vi "single fit V4 - rec.vi"(5 "cursor bracket: fragment  ref":refnum<vi>, 6 "main VI path":path, 7 "factor":dbl=7.0, 8 "pond":cdb[][](array[numeric]), 9 "wave packet":cdb[][](array[numeric]), 10 "omega map parameters":T2={"map method"=enum."less trivial", "2:window factor"=1, "left"=3.0, "right"=3.0, "omega"=3.0, "gamma"=3.0, "theta0"=3.0, "use points"=enum."decimated", "z(inf) method"=enum."median"}, 11 "single fit parameters":T3={"number of 2D grid points"=300, "# of points in pond"=339, "# of points in window"=10919, "decimation threshold"=1, "normalization factor"=0.029014793, "pond scale factor "=3.0, "normalized z"=[], "decimated z"=[], "decimated omega"=[], "omega in window"=[], "z in window"=[], "data center"=3.0+0.0i, "inverse"=[], "linear "=[], "omega around"=[], "phase around center"=[], "fit for phase around senter "=[], "three points"={[], []}, "max omega"=0.029014793, "min omega"=0.029014793}) -> (0 "lorentzian out":T5={"Amplitude"=-1.0311345636926572, "omega(0)"=-1.0311345636926572, "Gamma"=-1.0311345636926572, "phase"=-1.0311345636926572, "Q"=-1.0311345636926572, "Norm  Ampl"=-1.0311345636926572, "z (inf)"=-1.0311345636926572+0.0i, "4corners"={"z (-pi/2)"=-1.0311345636926572+0.5736824521422934i, "z(inf)"=-0.5200164984937075+1.0975277942502903i, "z (pi/2)"=-1.0311345636926572+0.5736824521422934i, "z center"=-0.5136528600391839+0.580046090596817i, "z(0)"=-0.5200164984937075+1.0975277942502903i, "radius"=-1.0311345636926572}} {"Q" format="%#_8f"; "phase" format="%#_6f"; "Gamma" format="%#_8f"; "omega(0)" format="%#_8f"}, 2 "omega map parameters out":T2={"map method"=enum."less trivial", "2:window factor"=1, "left"=3.0, "right"=3.0, "omega"=3.0, "gamma"=3.0, "theta0"=3.0, "use points"=enum."decimated", "z(inf) method"=enum."median"}, 3 "single fit parameters out":T3={"number of 2D grid points"=300, "# of points in pond"=339, "# of points in window"=10919, "decimation threshold"=1, "normalization factor"=0.029014793, "pond scale factor "=3.0, "normalized z"=[], "decimated z"=[], "decimated omega"=[], "omega in window"=[], "z in window"=[], "data center"=3.0+0.0i, "inverse"=[], "linear "=[], "omega around"=[], "phase around center"=[], "fit for phase around senter "=[], "three points"={[], []}, "max omega"=0.029014793, "min omega"=0.029014793}, 4 "complex region out":T4={"max re"=1.1965102077412717, "min re"=-1.8034897922587283, "max im"=1.1920568931854867, "min im"=-1.636084117505164, "delta re"=3.0, "delta im"=2.8281410106906506, "center re"=-0.3034897922587282, "delta  z"=3.0+2.8281410106906506i, "center im"=-0.2220136121598386, "center z"=-0.3034897922587282+2.8281410106906506i, "d im"=0.0, "d re"=0.0, "d z"=0.0+0.0i})   [LabVIEW 2010]
uses:
  lorentzian.ctl
  circle corners.ctl
  complex region.ctl
  single fit parameters.ctl
  omega map parameters.ctl
  cursor winow.ctl
  cursor window action.ctl
  peak - simple guess at omega.vi
  peak - less simple guess at omega.vi
  peak - fix phase.vi
  peak - fit phase around center.vi
  peak - geometry fit.vi
  find circle corners V3.vi
  peak - phase around center.vi
  peak - linear and inverse maps.vi
  peak - calculate lorentzian.vi
  index from range.vi
  <vilib>/Analysis/baseanly.llb/Mean.vi
  <vilib>/Analysis/baseanly.llb/Median.vi
  <vilib>/Analysis/2dsp.llb/Unwrap Phase.vi
  <vilib>/gmath/interp.llb/Interpolate 1D.vi
  <vilib>/gmath/NumericalOptimization/Nonlinear Curve Fit.vi
  <vilib>/gmath/NumericalOptimization/Nonlinear Curve Fit LM.vi
  <vilib>/Utility/error.llb/Clear Errors.vi
  <vilib>/Analysis/6fits.llb/Linear Fit.vi
panel:
  in  "cursor bracket in":T1={"left"=2044.0881763527054, "right "=2126.7657992565055, "center"=2085.4269878046052, "window"=82.67762290380006, "cursors"=[], "relative"=0, "absolute"=0, "fixed vertical offset"=2421.6740576496672, "vertical offset"=2421.6740576496672, "skew"=2421.6740576496672, "default window frac"=2421.6740576496672, "kind"=enum."fancy", "skew.left"=2.0, "skew.right"=0.0, "Plot ref"=refnum, "wing order"=enum."back"}
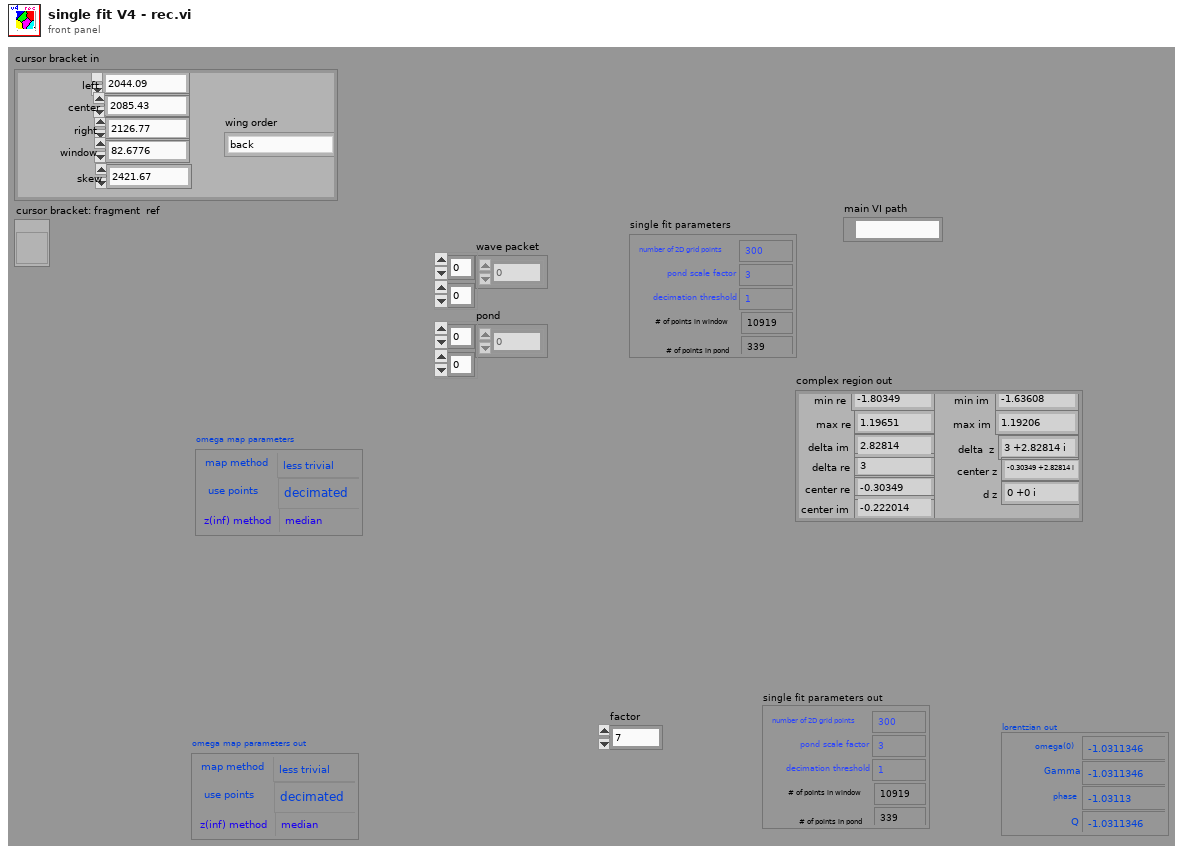
[diagram p1: front panel]
types:
  T1 = typedef "cursor winow.ctl" = cluster{"left":dbl, "right ":dbl, "center":dbl, "window":dbl, "cursors":i32[], "relative":i32, "absolute":i32, "fixed vertical offset":dbl, "vertical offset":dbl, "skew":dbl, "default window frac":dbl, "kind":enum16{"symmetric", "skewed", "fancy"}, "skew.left":dbl, "skew.right":dbl, "Plot ref":refnum<vi>, "wing order":enum16{"forw", "back"}}
  T2 = typedef "omega map parameters.ctl" = cluster{"map method":enum16{"simple", "less trivial", "around center", "geometry"}, "2:window factor":i32, "left":dbl, "right":dbl, "omega":dbl, "gamma":dbl, "theta0":dbl, "use points":enum16{"all in window", "decimated"}, "z(inf) method":enum16{"median", "method 2", "histogram"}}
  T3 = typedef "single fit parameters.ctl" = cluster{"number of 2D grid points":i32, "# of points in pond":i32, "# of points in window":i32, "decimation threshold":i32, "normalization factor":dbl, "pond scale factor ":dbl, "normalized z":cdb[], "decimated z":cdb[], "decimated omega":dbl[], "omega in window":dbl[], "z in window":cdb[], "data center":cdb, "inverse":cdb[], "linear ":cdb[], "omega around":dbl[], "phase around center":dbl[], "fit for phase around senter ":dbl[], "three points":cluster{dbl[], dbl[]}, "max omega":dbl, "min omega":dbl}
  T4 = typedef "complex region.ctl" = cluster{"max re":dbl, "min re":dbl, "max im":dbl, "min im":dbl, "delta re":dbl, "delta im":dbl, "center re":dbl, "delta  z":cdb, "center im":dbl, "center z":cdb, "d im":dbl, "d re":dbl, "d z":cdb}
  T5 = typedef "lorentzian.ctl" = cluster{"Amplitude":dbl, "omega(0)":dbl, "Gamma":dbl, "phase":dbl, "Q":dbl, "Norm  Ampl":dbl, "z (inf)":cdb, "4corners":T6}
  T6 = typedef "circle corners.ctl" = cluster{"z (-pi/2)":cdb, "z(inf)":cdb, "z (pi/2)":cdb, "z center":cdb, "z(0)":cdb, "radius":dbl}
  T7 = enum16{"simple", "less trivial", "around center", "geometry"}
  T8 = cluster{"left":dbl, "right ":dbl, "center":dbl, "window":dbl, "cursors":i32[], "relative":i32, "absolute":i32, "fixed vertical offset":dbl, "vertical offset":dbl, "skew":dbl, "default window frac":dbl, "kind":enum16{"symmetric", "skewed", "fancy"}, "skew.left":dbl, "skew.right":dbl, "Plot ref":refnum<vi>, "wing order":enum16{"forw", "back"}}
  T9 = typedef "cursor window action.ctl" = enum16{"balance", "h. offset change", "cursor moves", "change center", "change window", "init", "check", "reset", "set y to middle", "idle", "-write all Y", "-write left.X", "-write center.X", "-write right.X", "-write all X", "-change center", "-change window", "-change skew", "-read cursor 2", "-read cursor 1", "-read cursor 0", "-read all cursors", "-reset", "-read plot scale", "-set y to middle", "-Q: center.Y is visible", "-Q: window is visible", "-parse center.Y", "-right left from center", "-left move", "-right move", "-set center.Y", "-empty", "-set cursors to default", "-check", "-write center.Y", "-copy cursor 1", "-copy cursor 0", "-copy cursor 2", "move right", "move left", "shrink", "broaden", "skew up", "skew down", "-write plot scale", "zoom X"}
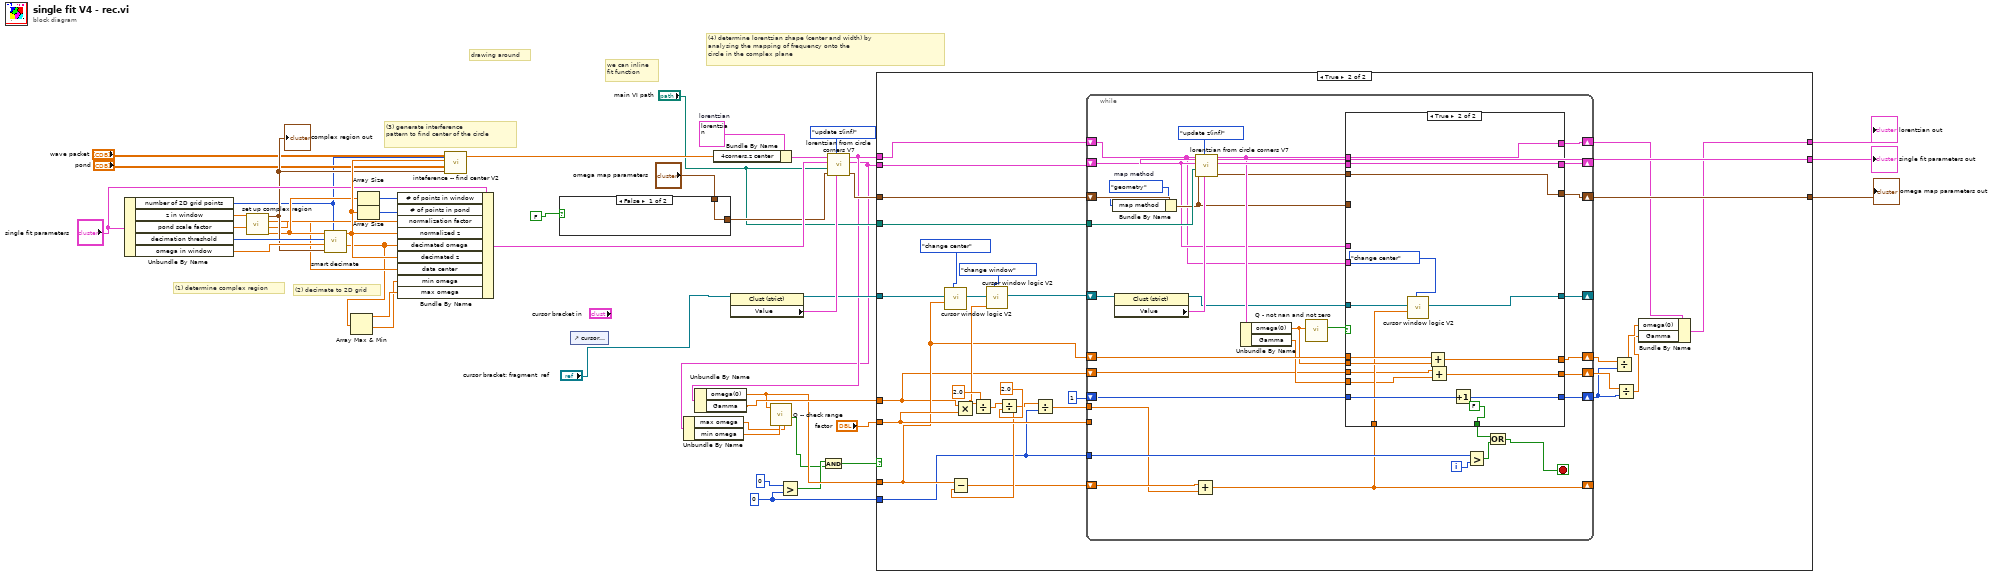
[diagram p0: block diagram]
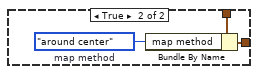
[diagram p2: hidden frame]
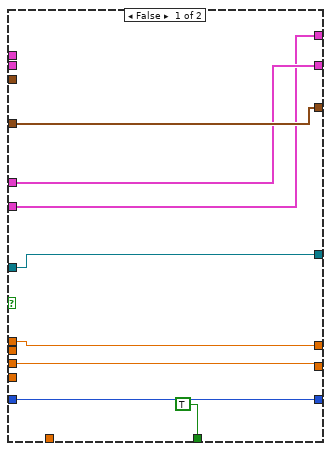
[diagram p4: hidden frame]
diagram:
  w7 = 0
  w30 = T5 {"Amplitude"=-1.0311345636926572, "omega(0)"=-1.0311345636926572, "Gamma"=-1.0311345636926572, "phase"=-1.0311345636926572, "Q"=-1.0311345636926572, "Norm  Ampl"=-1.0311345636926572, "z (inf)"=-1.0311345636926572+0.0i, "4corners"={"z (-pi/2)"=-1.0311345636926572+0.5736824521422934i, "z(inf)"=-0.5200164984937075+1.0975277942502903i, "z (pi/2)"=-1.0311345636926572+0.5736824521422934i, "z center"=-0.5136528600391839+0.580046090596817i, "z(0)"=-0.5200164984937075+1.0975277942502903i, "radius"=-1.0311345636926572}}  # lorentzian
  # "we can inline \nfit function"
  # "(4) determine lorentzian shape (center and width) by \nanalysing the mapping of frequency onto the\ncircle in the complex plane"
  # "(1) determine complex region"
  # "drawing around"
  # "(3) generate interference\npattern to find center of the circle"
  # "(2) decimate to 2D grid"
  n1 = Unbundle By Name("single fit parameters") -> ("number of 2D grid points"=w28:i32, "z in window"=w27:cdb[], "pond scale factor"=w40:dbl, "decimation threshold"=w46:i32, "omega in window"=w43:dbl[])
  n2 = call "set up complex region.vi"("scale factor"=w40, "z in window"=w27) -> ("z  normalized"=w38:cdb[], "normalization factor"=w37:dbl, "data center"=w36:cdb, "complex region"=w39:T4)  [unwired: 6 in]
  "complex region out" <- w39
  n3 = call "smart decimate .vi"("number of 2D grid points"=w28, "complex region"=w39, "omega in"=w43, "decimation threshold"=w46, "z in"=w38) -> ("decimated omega"=w13:dbl[], "decimated z"=w42:cdb[])  [unwired: 5 in]
  n4 = Array Max & Min(array=w13) -> (max value=w15:dbl, min value=w14:dbl)  [unwired: 2 out]
  n5 = Array Size(array=w38) -> (size(s)=w45:i32)
  n6 = Array Size(array=w42) -> (size(s)=w44:i32)
  n7 = Bundle By Name(cluster="single fit parameters", "# of points in window"=w45, "# of points in pond"=w44, "normalization factor"=w37, "normalized z"=w38, "decimated omega"=w13, "decimated z"=w42, "data center"=w36, "min omega"=w14, "max omega"=w15) -> (w35:T3)
  n8 = call "inteference -- find center V2.vi"("number of points"=w28, "complex region"=w39, "pond"="pond", "point sources"=w42, "wave packet"="wave packet") -> ("z (center)"=w34:cdb)  [unwired: 6 in]
  n9 = case shown="False" FALSE {
    tunnel: "omega map parameters" -> [w47 w50]
    tunnel: [w47 w49] -> w24
    frame False {
    }
    frame True {
      w48 = T7."around center"  # map method
      n10 = Bundle By Name(cluster=w50, "map method"=w48) -> (w49:T2)
    }
  }
  n11 = control-ref of="cursor bracket in"() -> ()  [unwired: 1 out]
  n12 = Bundle By Name(cluster=w30, "4corners.z center"=w34) -> (w29:T5)
  n13 = property class="Clust (strict)"(reference="cursor bracket: fragment  ref") -> (reference out=w19:refnum<vi>, "Value"=w26:T8)  [unwired: 1 in, 1 out]
  n14 = Greater?(x=0, y=w7) -> (0:w5:bool)
  n15 = call "lorentzian from circle corners V7.vi"("cursor bracket in"=w26, "update z(inf)"=enum16{"update z(inf)", "do not update z(inf)"}."update z(inf)", "omega map rameters in"=w24, "main VI  path"="main VI path", "parameters in: center detection"=w35, "lorentzian in"=w29) -> ("omega map parameters  out"=w18:T2, "parameters out  : center detection"=w12:T3, "lorentzian out"=w16:T5)  [unwired: 3 in]
  n16 = Unbundle By Name(w12) -> ("max omega"=w10:dbl, "min omega"=w11:dbl)
  n17 = Unbundle By Name(w16) -> ("omega(0)"=w8:dbl, "Gamma"=w9:dbl)
  n18 = call "Q -- check range.vi"("upper"=w10, "lower"=w11, "number"=w8) -> ("in range?"=w3:bool)  [unwired: 4 in, 4 out]
  n19 = And(x=w5, y=w3) -> (x .and. y?=w4:bool)
  n20 = case shown="True" w4 {
    tunnel: [w52 w83] -> w23
    tunnel: [w53 w63] -> w22
    tunnel: "main VI path" -> [_ w82]
    tunnel: [w51 w81] -> w20
    tunnel: w19 -> [_ w68]
    tunnel: w18 -> [w51 w80]
    tunnel: "factor" -> [_ w77]
    tunnel: w16 -> [w53 w79]
    tunnel: w12 -> [w52 w78]
    tunnel: w9 -> [_ w60]
    tunnel: w8 -> [_ w65]
    tunnel: w7 -> [_ w56]
    frame False {
    }
    frame True {
      n21 = call "cursor window logic V2.vi"("cursor window action"=cursor_window_action."change center", "center"=w65, "cursor window in"=w68) -> ("cursor window out"=w69:refnum<vi>)  [unwired: 7 in, 1 out]
      n22 = Multiply(x=w60, y=w77) -> (x*y=w66:dbl)
      n23 = Divide(x=w66, y=2.0) -> (x/y=w75:dbl)
      n24 = call "cursor window logic V2.vi"("cursor window action"=cursor_window_action."change window", "window"=w66, "cursor window in"=w69) -> ("cursor window out"=w67:refnum<vi>)  [unwired: 7 in, 1 out]
      n25 = Divide(x=w75, y=2.0) -> (x/y=w73:dbl)
      n26 = Subtract(x=w65, y=w73) -> (x-y=w72:dbl)
      n27 = Divide(x=w73, y=w56) -> (x/y=w71:dbl)
      n28 = while {
        shift-right: [w97] -> w83
        shift-left: w78 -> [w89]
        shift-right: [w99] -> w64
        shift-left: w79 -> [w88]
        tunnel: w82 -> [w117]
        shift-right: [w95] -> w81
        shift-left: w80 -> [w116]
        shift-right: [w92] -> _
        shift-left: w67 -> [w115]
        tunnel: w77 -> [_]
        tunnel: w56 -> [w111]
        shift-right: [w91] -> _
        shift-left: w72 -> [w110]
        tunnel: w71 -> [w109]
        shift-right: [w103] -> w58
        shift-left: 1 -> [w104]
        shift-right: [w100] -> w62
        shift-left: w65 -> [w102]
        shift-right: [w84] -> w59
        shift-left: w60 -> [w85]
        i -> [w114]
        stop <- w112 stop-if-true
        w107 = T7."geometry"  # map method
        n29 = Bundle By Name(cluster=w116, "map method"=w107) -> (w90:T2)
        n30 = property class="Clust (strict)"(reference=w115) -> (reference out=w93:refnum<vi>, "Value"=w106:T8)  [unwired: 1 in, 1 out]
        n31 = Add(x=w110, y=w109) -> (x+y=w91:dbl)
        n32 = call "lorentzian from circle corners V7.vi"("cursor bracket in"=w106, "update z(inf)"=enum16{"update z(inf)", "do not update z(inf)"}."update z(inf)", "omega map rameters in"=w90, "main VI  path"=w117, "parameters in: center detection"=w89, "lorentzian in"=w88) -> ("omega map parameters  out"=w94:T2, "parameters out  : center detection"=w96:T3, "lorentzian out"=w98:T5)  [unwired: 3 in]
        n33 = Unbundle By Name(w98) -> ("omega(0)"=w101:dbl, "Gamma"=w86:dbl)
        n34 = call "Q - not nan and not zero.vi"("Numeric"=w101) -> ("Boolean"=w105:bool)  [unwired: 10 in]
        n35 = case shown="True" w105 {
          tunnel: w104 -> [w120 w141]
          tunnel: [w120 w140] -> w103
          tunnel: w102 -> [w121 w139]
          tunnel: w101 -> [_ w138]
          tunnel: [w121 w137] -> w100
          tunnel: [w123 w136] -> w99
          tunnel: w98 -> [_ w136]
          tunnel: [w124 w135] -> w97
          tunnel: w96 -> [_ w135]
          tunnel: [w125 w134] -> w95
          tunnel: w94 -> [_ w134]
          tunnel: w93 -> [w119 w133]
          tunnel: [w119 w132] -> w92
          tunnel: w91 -> [_ w131]
          tunnel: w90 -> [w125 _]
          tunnel: w89 -> [w124 _]
          tunnel: w88 -> [w123 _]
          tunnel: [TRUE FALSE] -> w87
          tunnel: w86 -> [_ w129]
          tunnel: w85 -> [w118 w128]
          tunnel: [w118 w127] -> w84
          frame False {
          }
          frame True {
            n36 = call "cursor window logic V2.vi"("cursor window action"=cursor_window_action."change center", "center"=w131, "cursor window in"=w133) -> ("cursor window out"=w132:refnum<vi>)  [unwired: 7 in, 1 out]
            n37 = Add(x=w139, y=w138) -> (x+y=w137:dbl)
            n38 = Add(x=w128, y=w129) -> (x+y=w127:dbl)
            n39 = Increment(x=w141) -> (x+1=w140:i32)
          }
        }
        n40 = Greater?(x=w111, y=w114) -> (0:w113:bool)
        n41 = Or(x=w87, y=w113) -> (x .or. y?=w112:bool)
      }
      n42 = Divide(x=w62, y=w58) -> (x/y=w61:dbl)
      n43 = Divide(x=w59, y=w58) -> (x/y=w57:dbl)
      n44 = Bundle By Name(cluster=w64, "omega(0)"=w61, "Gamma"=w57) -> (w63:T5)
    }
  }
  "lorentzian out" <- w22
  "single fit parameters out" <- w23
  "omega map parameters out" <- w20
